vi "Cargo Solenid set.vi"(4 "SolenoidDevRef 4":T1={"DevStatus"={"status"=FALSE, "code"=0, "source"=""}, "Pneumatics Control Module"=0, "Forward Solenoid Channel"=enum."Invalid", "Reverse Solenoid Channel"=enum."Invalid"}, 5 "SolenoidDevRef":T1={"DevStatus"={"status"=FALSE, "code"=0, "source"=""}, "Pneumatics Control Module"=0, "Forward Solenoid Channel"=enum."Invalid", "Reverse Solenoid Channel"=enum."Invalid"}, 6 "SolenoidDevRef 3":T1={"DevStatus"={"status"=FALSE, "code"=0, "source"=""}, "Pneumatics Control Module"=0, "Forward Solenoid Channel"=enum."Invalid", "Reverse Solenoid Channel"=enum."Invalid"}, 7 "SolenoidDevRef 2":T1={"DevStatus"={"status"=FALSE, "code"=0, "source"=""}, "Pneumatics Control Module"=0, "Forward Solenoid Channel"=enum."Invalid", "Reverse Solenoid Channel"=enum."Invalid"}, 8 "Rocket_Shoot_Right_Solenoid_Position":bool, 9 "Rocket_Shoot_Left_Solenoid_Position":bool, 10 "Cargo_Shoot_Right_Solenoid_Position":bool, 11 "Cargo_Shoot_Left_Solenoid_Position":bool) -> ()   [LabVIEW 2018]
uses:
  <vilib>/Rock Robotics/WPI/Solenoid/WPI_SolenoidDevRef.ctl
  <vilib>/Rock Robotics/WPI/Solenoid/WPI_SolenoidChannel.ctl
  <vilib>/Rock Robotics/WPI/Solenoid/WPI_SolenoidValue.ctl
  <userlib>/836-Library/System/TDMS_V2/Support/TDMS_DevRef.ctl
  <userlib>/836-Library/System/TDMS_V2/Support/Logging_Settings.ctl
  <userlib>/836-Library/System/TDMS_V2/Support/Group_FIFO_Config.ctl
  <userlib>/836-Library/System/TDMS_V2/Support/Channel_FIFO_Config.ctl
  <vilib>/Rock Robotics/WPI/Solenoid/WPI_SolenoidSetEnum.vi
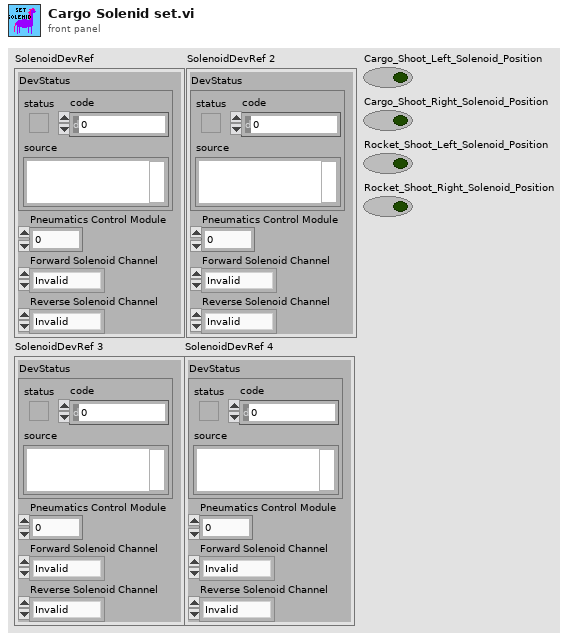
[diagram p1: front panel]
types:
  T1 = typedef "WPI_SolenoidDevRef.ctl" = cluster{"DevStatus":errorcluster, "Pneumatics Control Module":u8, "Forward Solenoid Channel":T2, "Reverse Solenoid Channel":T2}
  T2 = typedef "WPI_SolenoidChannel.ctl" = enum8{"Solenoid 0", "Solenoid 1", "Solenoid 2", "Solenoid 3", "Solenoid 4", "Solenoid 5", "Solenoid 6", "Solenoid 7", "Invalid"}
  T3 = typedef "WPI_SolenoidValue.ctl" = enum16{"Off", "On", "Forward", "Reverse"}
  T4 = typedef "TDMS_DevRef.ctl" = cluster{"Name":string, "File Ref":refnum<k34>, "Start Time":timestamp, "Logging Settings":T5, "Group FIFO Config":T6[], "Data To Write":refnum<data-value>, "semaphore":T8, "Ref Time Reset":refnum<k4>}
  T5 = typedef "Logging_Settings.ctl" = cluster{"Data Grab Period":dbl, "File Write Period":dbl, "Max Stored Size":dbl, "Burst Size":dbl}
  T6 = typedef "Group_FIFO_Config.ctl" = cluster{"Group":string, "Channels":T7[], "Channel Names":string[]}
  T7 = typedef "Channel_FIFO_Config.ctl" = cluster{"Channel":string, "FIFO":refnum<k33>}
  T8 = typedef "Semaphore RefNum" = refnum<k1>
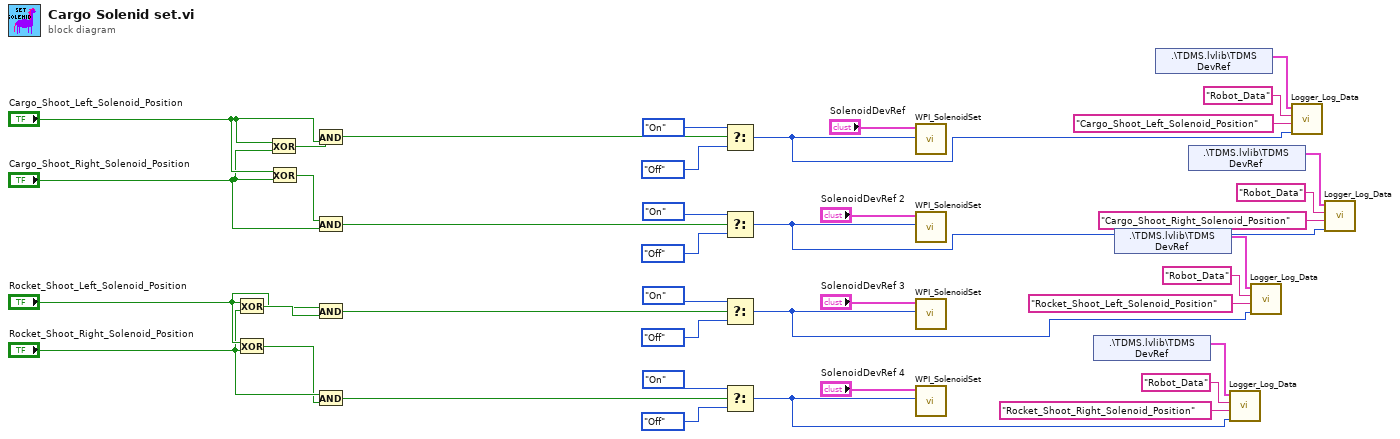
[diagram p0: block diagram]
diagram:
  n1 = Exclusive Or(1:"Rocket_Shoot_Right_Solenoid_Position", 2:"Rocket_Shoot_Left_Solenoid_Position") -> (0:w28:bool)
  n2 = Exclusive Or(1:"Rocket_Shoot_Right_Solenoid_Position", 2:"Rocket_Shoot_Left_Solenoid_Position") -> (0:w21:bool)
  n3 = Exclusive Or(1:"Cargo_Shoot_Right_Solenoid_Position", 2:"Cargo_Shoot_Left_Solenoid_Position") -> (0:w25:bool)
  n4 = Exclusive Or(1:"Cargo_Shoot_Right_Solenoid_Position", 2:"Cargo_Shoot_Left_Solenoid_Position") -> (0:w26:bool)
  n5 = And(x=w25, y="Cargo_Shoot_Left_Solenoid_Position") -> (x .and. y?=w4:bool)
  n6 = And(x=w26, y="Cargo_Shoot_Right_Solenoid_Position") -> (x .and. y?=w3:bool)
  n7 = And(x="Rocket_Shoot_Left_Solenoid_Position", y=w28) -> (x .and. y?=w2:bool)
  n8 = And(x="Rocket_Shoot_Right_Solenoid_Position", y=w21) -> (x .and. y?=w1:bool)
  n9 = Select(t=WPI_SolenoidValue."On" ("Value"), s=w4, f=WPI_SolenoidValue."Off" ("Value")) -> (s? t:f=w9:T3)
  n10 = Select(t=WPI_SolenoidValue."On" ("Value"), s=w3, f=WPI_SolenoidValue."Off" ("Value")) -> (s? t:f=w5:T3)
  n11 = Select(t=WPI_SolenoidValue."On" ("Value"), s=w2, f=WPI_SolenoidValue."Off" ("Value")) -> (s? t:f=w14:T3)
  n12 = Select(t=WPI_SolenoidValue."On" ("Value"), s=w1, f=WPI_SolenoidValue."Off" ("Value")) -> (s? t:f=w13:T3)
  n13 = call-poly <vilib>:"WPI_SolenoidSet.vi"("Value"=w9, "SolenoidDevRef"="SolenoidDevRef") -> ()  [unwired: 8 in, 2 out]
  n14 = call-poly <vilib>:"WPI_SolenoidSet.vi"("Value"=w5, "SolenoidDevRef"="SolenoidDevRef 2") -> ()  [unwired: 8 in, 2 out]
  n15 = call-poly <vilib>:"WPI_SolenoidSet.vi"("Value"=w14, "SolenoidDevRef"="SolenoidDevRef 3") -> ()  [unwired: 8 in, 2 out]
  n16 = call-poly <vilib>:"WPI_SolenoidSet.vi"("Value"=w13, "SolenoidDevRef"="SolenoidDevRef 4") -> ()  [unwired: 8 in, 2 out]
  n17 = shared-variable ".\\TDMS.lvlib\\TDMS DevRef"() -> (w19:T4)  [unwired: 1 in, 1 out]
  n18 = shared-variable ".\\TDMS.lvlib\\TDMS DevRef"() -> (w16:T4)  [unwired: 1 in, 1 out]
  n19 = shared-variable ".\\TDMS.lvlib\\TDMS DevRef"() -> (w11:T4)  [unwired: 1 in, 1 out]
  n20 = shared-variable ".\\TDMS.lvlib\\TDMS DevRef"() -> (w7:T4)  [unwired: 1 in, 1 out]
  n21 = call <userlib>:"Logger_Log_Data.vi"("Data"=w13, "Channel"="Rocket_Shoot_Right_Solenoid_Position", "Group"="Robot_Data", "TDMS DevRef"=w19) -> ()  [unwired: 7 in, 1 out]
  n22 = call <userlib>:"Logger_Log_Data.vi"("Data"=w14, "Channel"="Rocket_Shoot_Left_Solenoid_Position", "Group"="Robot_Data", "TDMS DevRef"=w16) -> ()  [unwired: 7 in, 1 out]
  n23 = call <userlib>:"Logger_Log_Data.vi"("Data"=w9, "Channel"="Cargo_Shoot_Left_Solenoid_Position", "Group"="Robot_Data", "TDMS DevRef"=w11) -> ()  [unwired: 7 in, 1 out]
  n24 = call <userlib>:"Logger_Log_Data.vi"("Data"=w5, "Channel"="Cargo_Shoot_Right_Solenoid_Position", "Group"="Robot_Data", "TDMS DevRef"=w7) -> ()  [unwired: 7 in, 1 out]
